vi "LV86_Morph_HitMiss.vi"(2 "Connectivity":enum16{"4", "6", "8"}(ring), 3 "Image in":T1 {"Dialogs" format="%.0b"}) -> (1 "Image out":T1 {"Dialogs" format="%.0b"})   [LabVIEW 2024]
doc: "This VI performs a Hit-or-Miss morphological operation on the input image. All pixel neighborhoods matching the given <B>connectivity</B> are kept. All others are removed. Input image must be binary."
uses:
  <userlib>/ImageProcessing/QTLIB_2595_LV86/QT_Image.ctl
  <vilib>/Analysis/2dsp.llb/2D Convolution (DBL).vi
  <vilib>/Analysis/NI_AALPro.lvlib
panel:
  # "This VI performs a Hit-or-Miss morphological \noperation on the input image.  All pixel neighborhoods \nmatching the given connectivity are kept.  All \nothers are removed.  Input image must be binary."
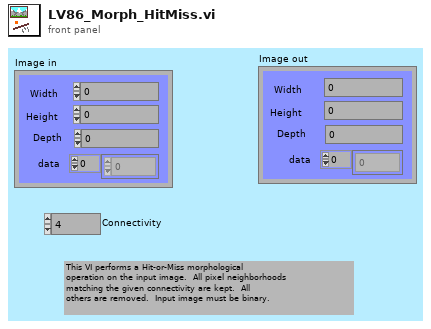
[diagram p1: front panel]
types:
  T1 = typedef "QT_Image.ctl" = cluster{"Width":i32, "Height":i32, "Depth":i32, "data":u8[], "Compressed data":u8[], "Color table":u32[], "Duration":i32, "Options":i32, "Timestamp":i32, "ID":i32, "Reserved":i32, "Dialogs":u32}
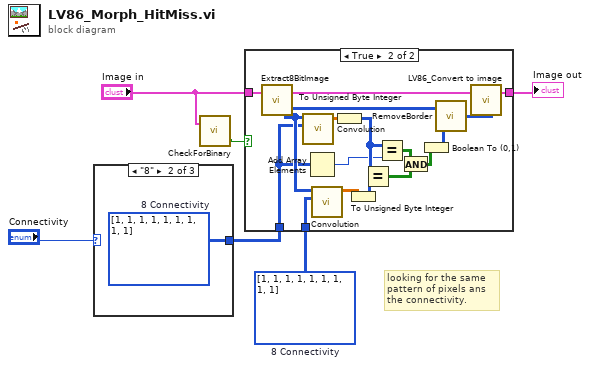
[diagram p0: block diagram]
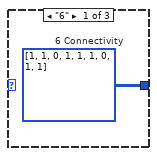
[diagram p3: hidden frame]
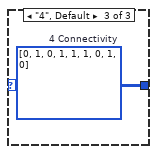
[diagram p4: hidden frame]
diagram:
  w1 = u8[][] [[1, 1, 1], [1, 1, 1], [1, 1, 1]]  # 8 Connectivity
  # "looking for the same \npattern of pixels ans\nthe connectivity."
  n1 = case shown="\"8\"" "Connectivity" {
    tunnel: [w7 w8 w9] -> w4
    frame "6" {
      w7 = u8[][] [[1, 1, 0], [1, 1, 1], [0, 1, 1]]  # 6 Connectivity
    }
    frame "8" {
      w8 = u8[][] [[1, 1, 1], [1, 1, 1], [1, 1, 1]]  # 8 Connectivity
    }
    frame "4", Default {
      w9 = u8[][] [[0, 1, 0], [1, 1, 1], [0, 1, 0]]  # 4 Connectivity
    }
  }
  n2 = call <userlib>:"CheckForBinary.vi"("Image in"="Image in") -> ("Success?"=w6:bool)  [unwired: 2 out]
  n3 = case shown="True" w6 {
    tunnel: "Image in" -> [w10 w25]
    tunnel: [w10 w24] -> w2
    tunnel: w4 -> [_ w15]
    tunnel: w1 -> [_ w20]
    frame False {
    }
    frame True {
      n4 = call <userlib>:"Extract8BitImage.vi"("Image in"=w25) -> ("Intensity Graph"=w21:u8[][], "Image out"=w26:T1)  [unwired: 1 in]
      n5 = call-poly <vilib>:"Convolution.vi"("Y"=w15, "X"=w21) -> ("X * Y"=w22:dbl[][])  [unwired: 2 in, 7 out]
      n6 = Add Array Elements(numeric array=w15) -> (sum=w14:u8)
      n7 = call-poly <vilib>:"Convolution.vi"("Y"=w20, "X"=w21) -> ("X * Y"=w19:dbl[][])  [unwired: 2 in, 7 out]
      n8 = To Unsigned Byte Integer(number=w22) -> (unsigned 8bit integer=w16:u8[][])
      n9 = To Unsigned Byte Integer(number=w19) -> (unsigned 8bit integer=w17:u8[][])
      n10 = Equal?(x=w16, y=w17) -> (x = y?=w12:bool[][])
      n11 = Equal?(x=w16, y=w14) -> (x = y?=w11:bool[][])
      n12 = And(x=w11, y=w12) -> (x .and. y?=w18:bool[][])
      n13 = Boolean To (0,1)(Boolean=w18) -> (0, 1=w13:i16[][])
      n14 = call <userlib>:"RemoveBorder.vi"("Larger Image"=w13, "Original Image"=w21) -> ("Subset"=w23:u8[][])
      n15 = call <userlib>:"LV86_Convert to image.vi"("Intensity Graph"=w23, "Image In"=w26) -> ("Image Out"=w24:T1)  [unwired: 1 in]
    }
  }
  "Image out" <- w2
